vi "Ping.vi"(6 "Response Timeout(100ms)":i32=100, 7 "TcpRouter-Client in":refnum<class "TcpRouter-Client.lvclass">, 8 "error in (no error)":errorcluster, 9 "TCP Wait If need connection(ms)":i32=5) -> (0 "error out":errorcluster, 2 "Server Ready?":bool)   [LabVIEW 2020, in "CSM-TCP-Router.lvlib" / "TcpRouter-Client.lvclass"]
uses:
  TcpRouter-Client.lvclass
  _support/tcp-msg type.ctl
  f32241c3-0036-4787-bc41-e9c1f987f5e1.vi
  <userlib>/_NEVSTOP/Communicable State Machine(CSM)/AdvanceAPI/CSM - Revert Arguments-Safe String.vi
  <userlib>/_NEVSTOP/Communicable State Machine(CSM)/_Support/Common/Trim Single line Text.vi
  <userlib>/_NEVSTOP/Communicable State Machine(CSM)/AdvanceAPI/CSM - Keywords.vi
  TcpRouter-Client.lvclass/TcpRouter-Client.ctl
  CSM-TCP-Router.lvlib
  <userlib>/_NEVSTOP/Communicable State Machine(CSM)/Communicable State Machine.lvlib
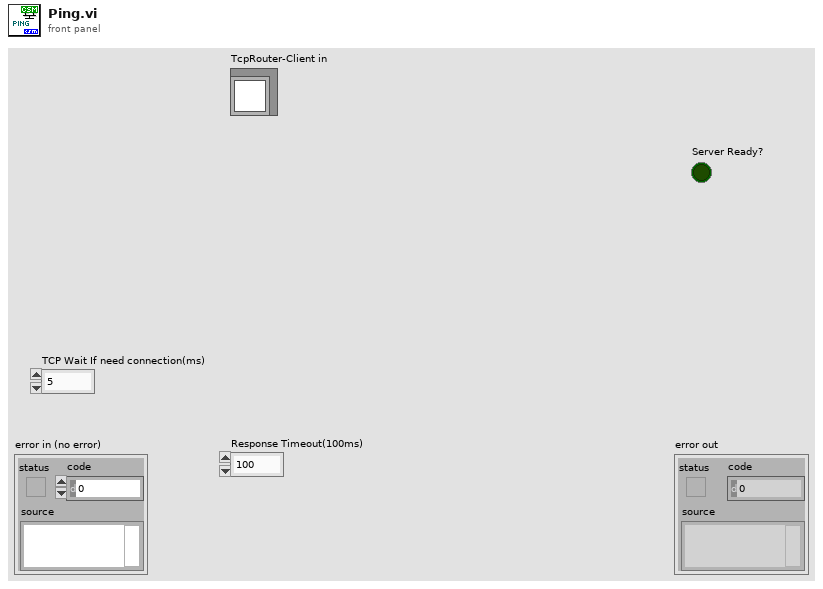
[diagram p1: front panel]
types:
  T1 = typedef "CSM-TCP-Router.lvlib/tcp-msg type.ctl" = enum8{"info", "error", "cmd", "cmd-resp", "resp", "async-resp", "status", "interrupt"}
  T2 = typedef "CSM-TCP-Router.lvlib/TcpRouter-Client.lvclass/Def-TCP-Router REQ-REP.ctl" = cluster{"REQ-REP":refnum<k5>}
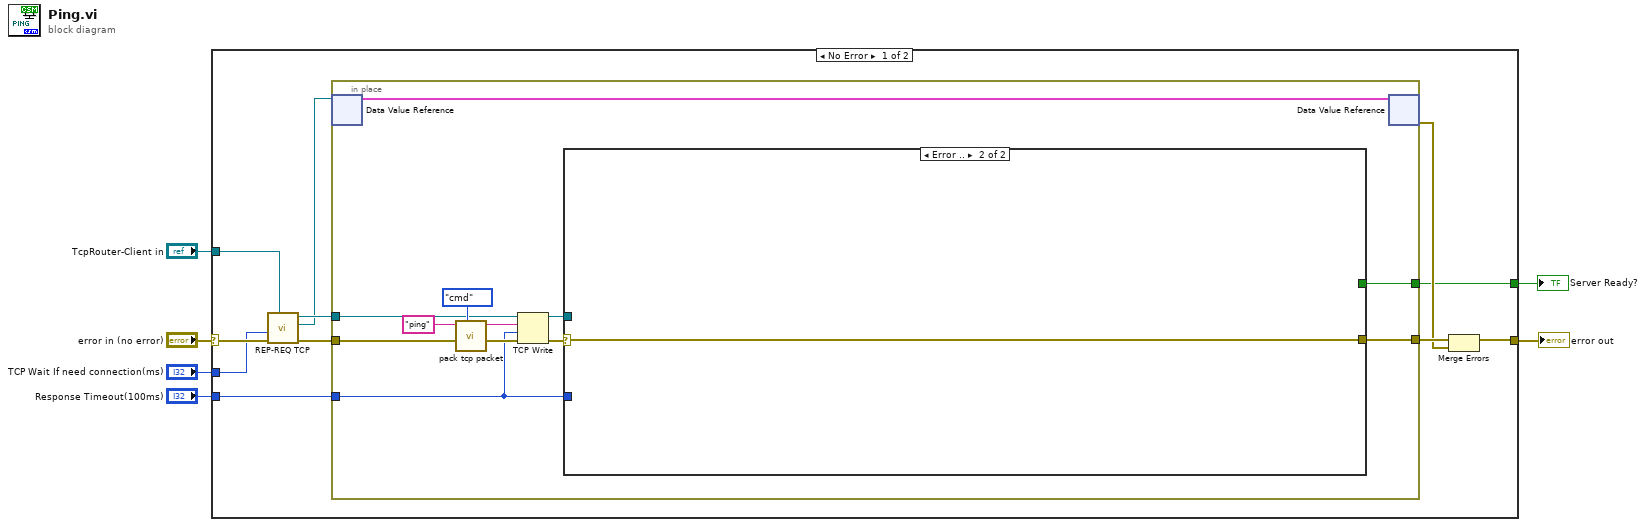
[diagram p0: block diagram]
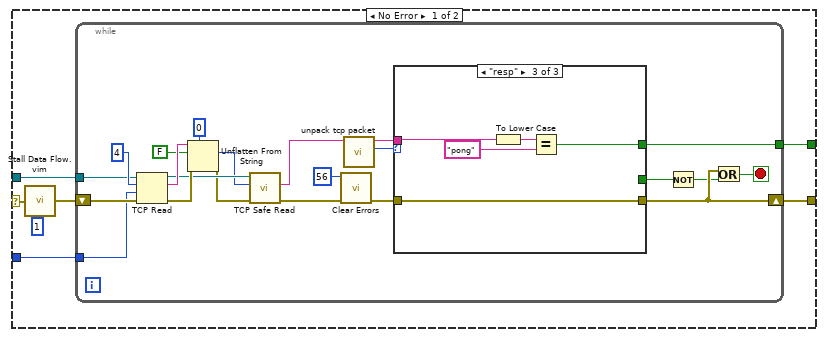
[diagram p2: hidden frame]
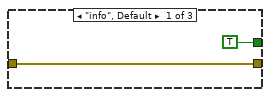
[diagram p3: hidden frame]
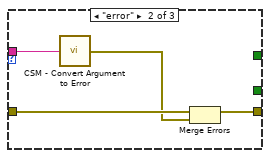
[diagram p4: hidden frame]
diagram:
  n1 = case shown="No Error" "error in (no error)" {
    selector: "error in (no error)" -> [w17 w70]
    tunnel: [w10 w70] -> w5
    tunnel: "TcpRouter-Client in" -> [w16 _]
    tunnel: "Response Timeout(100ms)" -> [w12 _]
    tunnel: [w8 _] -> w2
    tunnel: "TCP Wait If need connection(ms)" -> [w7 _]
    frame No Error {
      n2 = call "REP-REQ TCP.vi"("TcpRouter-Client in"=w16, "error in (no error)"=w17, "timeout ms (minus value for input)"=w7) -> ("error out"=w15:errorcluster, "REQ-REP"=w11:refnum<data-value>, "connection ID"=w14:refnum<k5>)  [unwired: 6 in]
      n3 = in-place {
        in-place-border: w15 -> [w26]
        in-place-border: w14 -> [w25]
        in-place-border: [w22] -> w13
        in-place-border: w12 -> [w21]
        in-place-border: [w18] -> w8
        n4 = in-place-dvr #1(w11) -> (w20:T2)  [unwired: 1 out]
        n5 = call "pack tcp packet.vi"("tcp-message-type"=tcp-msg_type."cmd", "String"="ping") -> ("TCP Pack"=w28:string)  [unwired: 9 in]
        n6 = TCP Write(connection ID=w25, data in=w28, error in (no error)=w26, 9:w21) -> (connection ID out=w23:refnum<k5>, error out=w24:errorcluster)  [unwired: 1 out]
        n7 = case shown="Error .." w24 {
          selector: w24 -> [w35 w69]
          tunnel: w23 -> [w33 _]
          tunnel: [w31 w69] -> w22
          tunnel: w21 -> [w30 _]
          tunnel: [w29 _] -> w18
          frame No Error {
            n8 = call "Stall Data Flow.vim"("value in"=w35, "milliseconds to wait"=u32 1) -> ("value out"=w32:errorcluster)  [unwired: 1 out]
            n9 = while {
              tunnel: w33 -> [w48]
              shift-right: [w43] -> w31
              shift-left: w32 -> [w47]
              tunnel: w30 -> [w42]
              tunnel: [w38] -> w29
              stop <- w41 stop-if-true
              n10 = TCP Read(connection ID=w48, bytes to read=4, error in (no error)=w47, 9:w42) -> (connection ID out=w55:refnum<k5>, data out=w56:string, error out=w57:errorcluster)  [unwired: 1 in]
              n11 = Unflatten From String(type=0, binary string=w56, data includes array or string size? (T)=FALSE, error in (no error)=w57) -> (value=w53:i32, error out=w52:errorcluster)  [unwired: 2 out]
              n12 = call "TCP Safe Read.vi"("error in (no error)"=w52, "bytes to read"=w53, "TCP Network Connection in"=w55) -> ("error out"=w45:errorcluster, "String"=w54:string)  [unwired: 6 in, 1 out]
              n13 = call <vilib>:"Clear Errors.vi"("error in (no error)"=w45, "specific error code to clear (0: all)"=56) -> ("error out"=w37:errorcluster)  [unwired: 4 in, 1 out]
              n14 = call "unpack tcp packet.vi"("TCP Pack"=w54) -> ("tcp-message-type"=w46:T1, "String"=w44:string)  [unwired: 9 in]
              n15 = case shown="\"resp\"" w46 {
                tunnel: w37 -> [w59 w63 w68]
                tunnel: [w59 w61 w68] -> w43
                tunnel: w44 -> [_ w62 w67]
                tunnel: [TRUE _ _] -> w40
                tunnel: [_ _ w64] -> w38
                frame "info", Default {
                }
                frame "error" {
                  n16 = call <userlib>:"CSM - Convert Argument to Error.vi"("Argument"=w62) -> ("error"=w60:errorcluster)  [unwired: 4 in]
                  n17 = Merge Errors(w63, w60) -> (w61:errorcluster)
                }
                frame "resp" {
                  n18 = To Lower Case(string=w67) -> (all lower case string=w65:string)
                  n19 = Equal?(x=w65, y="pong") -> (x = y?=w64:bool)
                }
              }
              n20 = Not(x=w40) -> (.not. x?=w39:bool)
              n21 = Or(x=w43, y=w39) -> (x .or. y?=w41:bool)
            }
          }
          frame Error {
          }
        }
        n22 = in-place-dvr #1(w20) -> (w9:errorcluster)  [unwired: 1 out]
      }
      n23 = Merge Errors(w13, w9) -> (w10:errorcluster)
    }
    frame Error {
    }
  }
  "error out" <- w5
  "Server Ready?" <- w2
